vi "Voltage input module.vi"(0 "Device Select":string(combo)="None", 1 "Init":bool, 2 "Exec":bool, 3 "finish up":bool, 5 "Input Control pipe":T2, 11 "Error In":errorcluster, 12 "Average":i32=1) -> (4 "current Control pipe":T2, 6 "output cluster":T1, 15 "Error out":errorcluster)   [LabVIEW 2023]
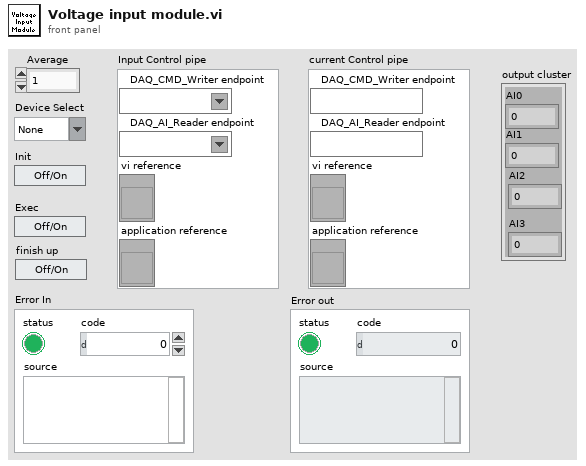
[diagram p1: front panel]
types:
  T1 = cluster{"AI0":dbl, "AI1":dbl, "AI2":dbl, "AI3":dbl}
  T2 = cluster{"DAQ_CMD_Writer endpoint":refnum<k21>, "DAQ_AI_Reader endpoint":refnum<k21>, "vi reference":refnum<vi>, "application reference":refnum<vi>}
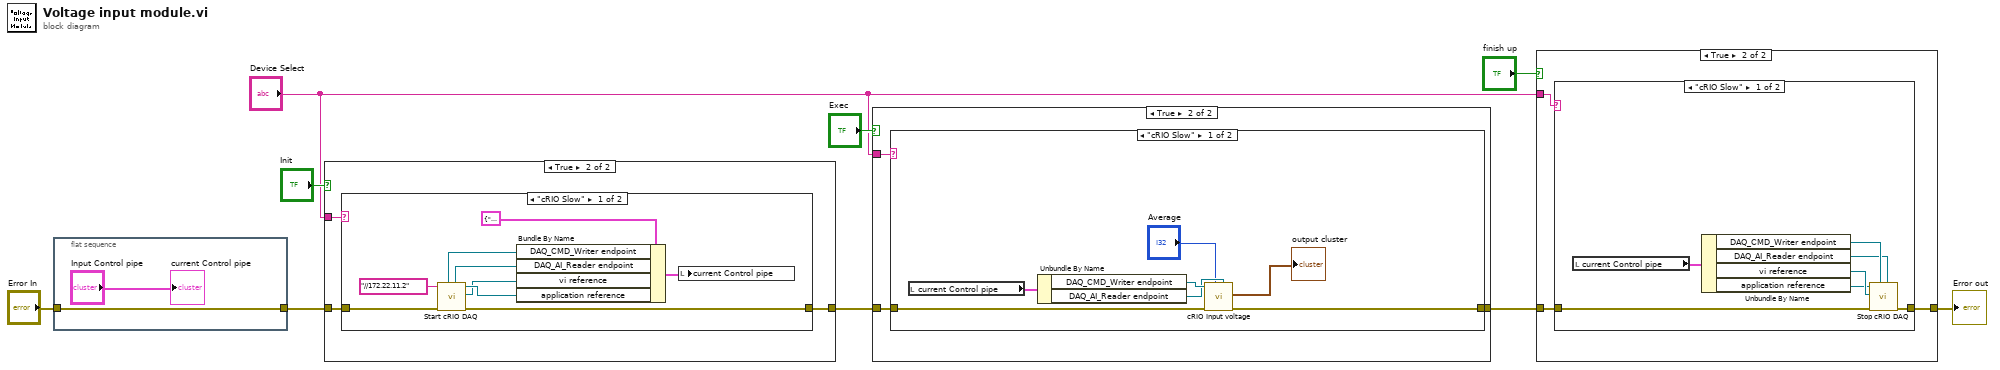
[diagram p0: block diagram]
diagram:
  n1 = flat-sequence {
    tunnel: "Error In" -> [w11]
    tunnel: [w11] -> w1
    frame #0 {
      "current Control pipe" <- "Input Control pipe"
    }
  }
  n2 = case shown="True" "Init" {
    tunnel: w1 -> [w12 w14]
    tunnel: [w12 w13] -> w6
    tunnel: "Device Select" -> [_ w15]
    frame False {
    }
    frame True {
      n3 = case shown="\"cRIO Slow\"" w15 {
        tunnel: w14 -> [w24 w25]
        tunnel: [w23 w25] -> w13
        frame "cRIO Slow" {
          n4 = call "Start cRIO DAQ.vi"("error in (no error)"=w24, "cRIO IP"="//172.22.11.2") -> ("error out"=w23:errorcluster, "vi reference"=w17:refnum<vi>, "application reference"=w18:refnum<vi>, "DAQ_AI_Reader endpoint"=w19:refnum<k21>, "DAQ_CMD_Writer endpoint"=w20:refnum<k21>)  [unwired: 5 in]
          n5 = Bundle By Name(cluster=T2 {"DAQ_CMD_Writer endpoint"="", "DAQ_AI_Reader endpoint"="", "vi reference"=refnum, "application reference"=refnum} ("current Control pipe"), "DAQ_CMD_Writer endpoint"=w20, "DAQ_AI_Reader endpoint"=w19, "vi reference"=w17, "application reference"=w18) -> (w16:T2)
          n6 = local write "current Control pipe"(w16) -> ()
        }
        frame "None", Default {
        }
      }
    }
  }
  n7 = case shown="True" "Exec" {
    tunnel: w6 -> [w26 w28]
    tunnel: [w26 w27] -> w5
    tunnel: "Device Select" -> [_ w29]
    frame False {
    }
    frame True {
      n8 = case shown="\"cRIO Slow\"" w29 {
        tunnel: w28 -> [w36 w37]
        tunnel: [w35 w37] -> w27
        frame "cRIO Slow" {
          n9 = local read "current Control pipe"() -> (w34:T2)
          n10 = Unbundle By Name(w34) -> ("DAQ_CMD_Writer endpoint"=w33:refnum<k21>, "DAQ_AI_Reader endpoint"=w32:refnum<k21>)
          n11 = call "cRIO Input voltage.vi"("DAQ_AI_Reader endpoint"=w32, "Average"="Average", "error in (no error)"=w36, "DAQ_CMD_Writer endpoint"=w33) -> ("error out"=w35:errorcluster, "output cluster"=→"output cluster":T1)  [unwired: 5 in, 1 out]
        }
        frame "None", Default {
        }
      }
    }
  }
  n12 = case shown="True" "finish up" {
    tunnel: w5 -> [w38 w40]
    tunnel: [w38 w39] -> w4
    tunnel: "Device Select" -> [_ w41]
    frame False {
    }
    frame True {
      n13 = case shown="\"cRIO Slow\"" w41 {
        tunnel: w40 -> [w48 w49]
        tunnel: [w47 w49] -> w39
        frame "cRIO Slow" {
          n14 = local read "current Control pipe"() -> (w46:T2)
          n15 = Unbundle By Name(w46) -> ("DAQ_CMD_Writer endpoint"=w45:refnum<k21>, "DAQ_AI_Reader endpoint"=w44:refnum<k21>, "vi reference"=w43:refnum<vi>, "application reference"=w42:refnum<vi>)
          n16 = call "Stop cRIO DAQ.vi"("DAQ_AI_Reader endpoint"=w44, "DAQ_CMD_Writer endpoint"=w45, "error in (no error)"=w48, "VI reference"=w43, "application reference"=w42) -> ("error out"=w47:errorcluster)  [unwired: 6 in]
        }
        frame "None", Default {
        }
      }
    }
  }
  "Error out" <- w4
